vi "Mcp2210 Read EE Prom.vi"(8 "error in (no error)":errorcluster, 10 "address":u8, 11 "handle":i32) -> (0 "error out":errorcluster, 2 "Value":u8, 3 "handle out":i32)   [LabVIEW 2015, in "mcp2210.lvlib"]
doc: "Read the byte at the EEPROM memory address provided as parameter.\nThe function returns negative error code in case of failure.\nThe EEPROM size is 256 bytes.\nParameters:\nInputs:\n- void *handle - The pointer to the USB device handle. Cannot be NULL.\n- unsigned char address - the EEPROM location to be read.\nOutputs:\n- unsigned char *pcontent - the value stored at the EEPROM address, if the function returns\nE_SUCCESS. In case of failure, *pcontent is not changed.\nThe parameter cannot be NULL.\nReturns:\n- 0 for success: E_SUCCESS\n- negative error code: E_ERR_NULL, E_ERR_INVALID_HANDLE_VALUE\nE_ERR_HID_TIMEOUT, E_ERR_HID_RW_FILEIO, E_ERR_UNKOWN_ERROR\nE_ERR_CMD_ECHO, E_ERR_CMD_FAILED\n\nMCP2210_DLL_UM_API int __stdcall Mcp2210_ReadEEProm(void *handle, unsigned char address, unsigned char *pcontent);"
uses:
  <userlib>/mcp2210/mcp2210.lvlib
  <userlib>/mcp2210/mcp2210_dll_um_x86.dll
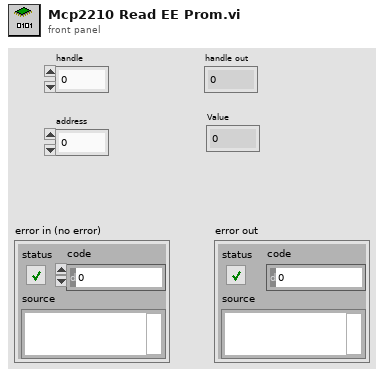
[diagram p1: front panel]
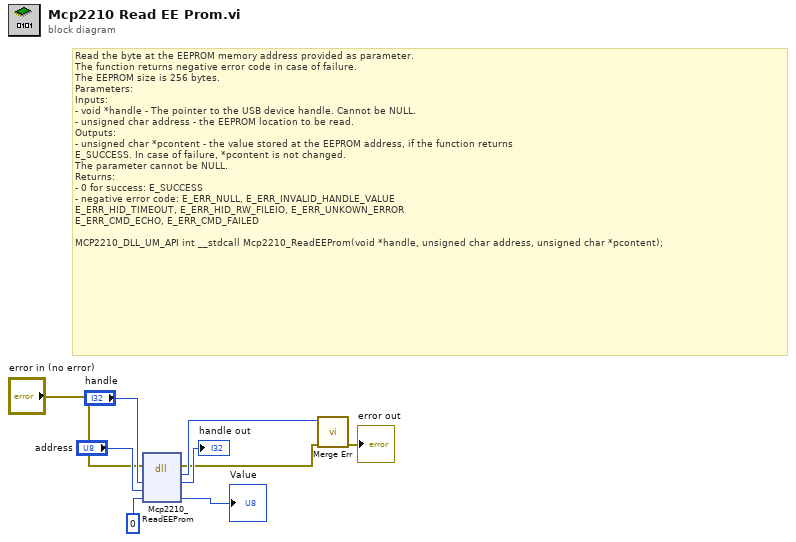
[diagram p0: block diagram]
diagram:
  # "Read the byte at the EEPROM memory address provided as parameter.\nThe function returns negative error code in case of failure.\nThe EEPROM size is 256 bytes.\nParameters:\nInputs:\n- void *handle - The pointer to the USB device handle. Cannot be NULL.\n- unsigned char address - the EEPROM location to be read.\nOutputs:\n- unsigned char *pcontent - the value stored at the EEPROM address, if the function returns\nE_SUCCESS. In case of failure, *pcontent is not changed.\nThe parameter cannot be NULL.\nReturns:\n- 0 for success: E_SUCCESS\n- negative error code: E_ERR_NULL, E_ERR_INVALID_HANDLE_VALUE\nE_ERR_HID_TIMEOUT, E_ERR_HID_RW_FILEIO, E_ERR_UNKOWN_ERROR\nE_ERR_CMD_ECHO, E_ERR_CMD_FAILED\n\nMCP2210_DLL_UM_API int __stdcall Mcp2210_ReadEEProm(void *handle, unsigned char address, unsigned char *pcontent);"
  n1 = dll-call lib="D:/LabVIEW 2015/user.lib/mcp2210/mcp2210_dll_um_x86.*" fn="Mcp2210_ReadEEProm"(error in="error in (no error)", "handle"="handle", "address"="address", "pcontent"=u8 0) -> (error out=w5:errorcluster, "return type"=w6:i32, "handle"=→"handle out":i32, "pcontent"=→"Value":u8)  [unwired: 3 in, 1 out]
  n2 = call <userlib>:"Merge Err.vi"("error in (no error)"=w5, "return type"=w6) -> ("error out"=→"error out":errorcluster)  [unwired: 9 in]
